vi "LLM_Basic.vi"() -> ()   [LabVIEW 2018]
doc: "This example demonstrates how to use OpenVINO to infer DeepSeek in LabVIEW to enable real-time streaming, processing, and display of data (e.g., text)."
uses:
  vi.lib/VIRobotics/OpenVINO_GenAI/LLMPipeline/Generate_Basic.vi
  vi.lib/VIRobotics/OpenVINO_GenAI/LLMPipeline/LLMPipeline.lvclass
panel:
  in  "device_name":string(combo)="CPU"
  in  "model_folder":path=path "D:/code/llm/deepseek/Deepseek-R1-1.5B-Instruct-int4-ov"
  in  "Prompt":string
  out "Answer":string
  # "Overview: This example demonstrates how to use OpenVINO to infer  DeepSeek in LabVIEW to enable real-time streaming, processing, and display of data (e.g., text). \nRequirements: Windows.\nInstructions: \n1.Select the model folder to use.\n2.Enter the prompt keywords\n3.Run the VI."
  # "LLM Stream Example for LabVIEW"
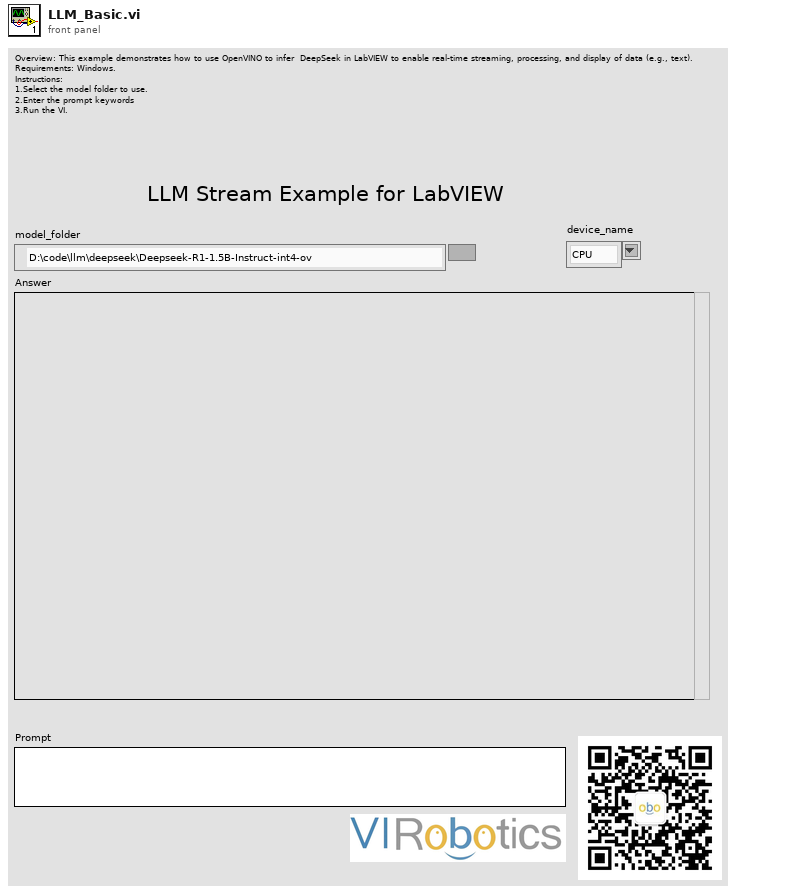
[diagram p1: front panel]
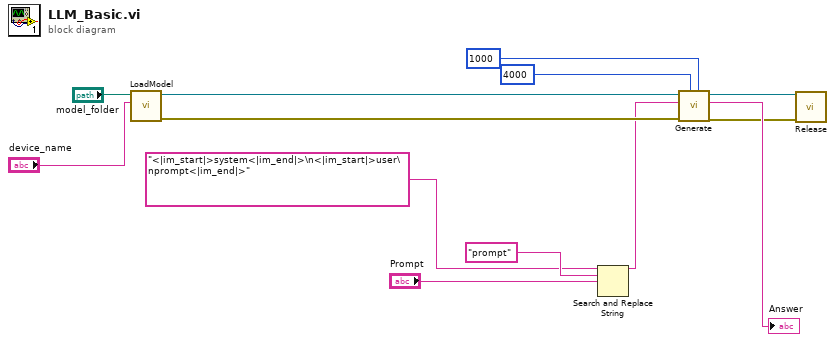
[diagram p0: block diagram]
diagram:
  n1 = call "LoadModel.vi"("device"="device_name", "path"="model_folder") -> ("error out"=w12:errorcluster, "LLMPipeline out"=w13:refnum<class "LLMPipeline.lvclass">)  [unwired: 8 in]
  n2 = Search and Replace String(input string="<|im_start|>system<|im_end|>\n<|im_start|>user\nprompt<|im_end|>", search string="prompt", replace string="Prompt") -> (result string=w5:string)  [unwired: 5 in, 3 out]
  n3 = call-poly "Generate.vi"("max_length"=1000, "max_new_tokens"=4000, "error in (no error)"=w12, "prompt"=w5, "LLMPipeline in"=w13) -> ("error out"=w2:errorcluster, "result"=→"Answer":string, "LLMPipeline out"=w3:refnum<class "LLMPipeline.lvclass">)  [unwired: 4 in]
  n4 = call "Release.vi"("error in (no error)"=w2, "LLMPipeline in"=w3) -> ()  [unwired: 8 in, 2 out]
